vi "Stop.vi"(8 "error in (no error)":errorcluster, 10 "Message in":refnum<class "StopMessage.lvclass">, 11 "DAQMH121119OrcaFlash in":refnum<class "DAQOrcaFlash.lvclass">) -> (0 "error out":errorcluster, 3 "DAQMH121119OrcaFlash out":refnum<class "DAQOrcaFlash.lvclass">)   [LabVIEW 2012, in "DAQOrcaFlash.lvclass"]
doc: "This member function is called when the statemachine in the run.vi receives an 'stop' command. It relays the message to all observers of the component.\n\nOverride this member function in your derived class if you need additional stop functionality (but don't forget to call the parent method)."
uses:
  DAQOrcaFlash.lvclass
  <vilib>/Distrio/Murmex/StopMessage/StopMessage.lvclass
  <vilib>/Distrio/Murmex/Murmex/Murmex.lvclass
  trigger_source.ctl
  trigger_mode.ctl
  DAQOrcaFlash.lvclass/DAQOrcaFlash.ctl
  imaging_mode.ctl
panel:
  # "This method is called when the STOP\ntrigger is sent. \n\nOverride this method when your component needs to\nrespond to this trigger. \n\nCall parent for proper implementation"
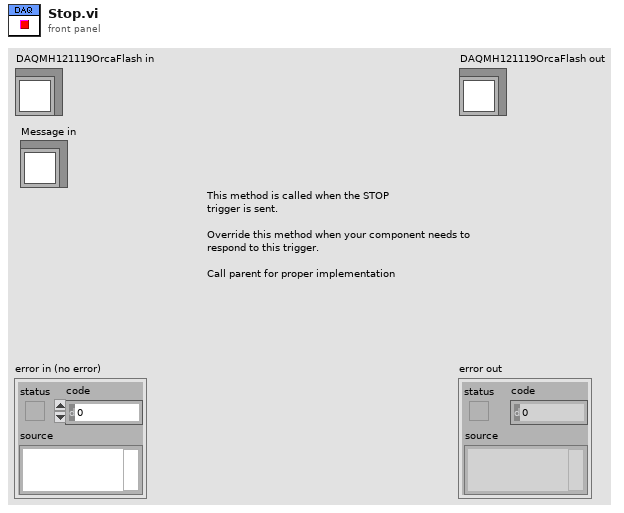
[diagram p1: front panel]
types:
  T1 = typedef "DAQOrcaFlash.lvclass/imaging_mode.ctl" = enum16{"focus mode", "single sweep"}
  T2 = typedef "DAQOrcaFlash.lvclass/trigger_mode.ctl" = sgl
  T3 = typedef "DAQOrcaFlash.lvclass/trigger_source.ctl" = sgl
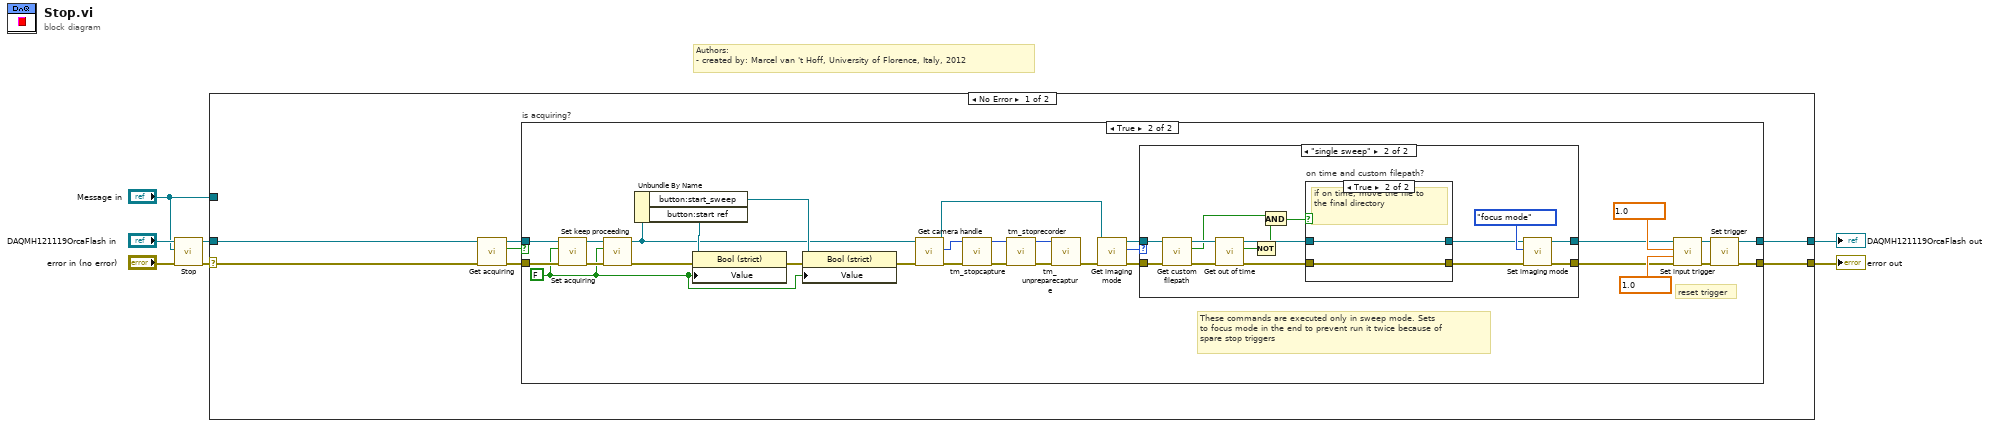
[diagram p0: block diagram]
diagram:
  # "Authors: \n- created by: Marcel van 't Hoff, University of Florence, Italy, 2012"
  n1 = call-parent "Stop.vi"("error in (no error)"="error in (no error)", "Message in"="Message in", "Murmex in"="DAQMH121119OrcaFlash in") -> ("error out"=w5:errorcluster, "Murmex out"=w2:refnum<class "DAQOrcaFlash.lvclass">)  [unwired: 7 in]
  n2 = case shown="No Error" w5 {
    selector: w5 -> [w9 w68]
    tunnel: [w11 w68] -> w4
    tunnel: [w10 w69] -> w3
    tunnel: w2 -> [w8 w69]
    tunnel: "Message in" -> [_ _]
    frame No Error {
      n3 = call "Get acquiring.vi"("error in (no error)"=w9, "DAQMH121119OrcaFlash in"=w8) -> ("error out"=w13:errorcluster, "is acquiring?"=w12:bool, "DAQMH121119OrcaFlash out"=w14:refnum<class "DAQOrcaFlash.lvclass">)  [unwired: 7 in]
      n4 = case "is acquiring?" shown="True" w12 {
        tunnel: [w15 w17] -> w10
        tunnel: [w16 w19] -> w11
        tunnel: w14 -> [w15 w44]
        tunnel: w13 -> [w16 w43]
        frame False {
        }
        frame True {
          w21 = T2 1.0 items=["Normal"=1.0, "Start"=6.0] ("Trigger mode")
          w22 = T3 1.0 items=["Internal"=1.0, "External"=2.0, "Software"=3.0] ("Trigger source")
          w25 = FALSE ("is acquiring?")
          # "reset trigger"
          # "These commands are executed only in sweep mode. Sets\nto focus mode in the end to prevent run it twice because of \nspare stop triggers"
          n5 = call "Set acquiring.vi"("error in (no error)"=w43, "is acquiring?"=w25, "DAQMH121119OrcaFlash in"=w44) -> ("error out"=w45:errorcluster, "DAQMH121119OrcaFlash out"=w27:refnum<class "DAQOrcaFlash.lvclass">)  [unwired: 7 in]
          n6 = call-dynamic "Set keep proceeding.vi"("error in (no error)"=w45, "keep proceeding?"=w25, "DAQOrcaFlash in"=w27) -> ("error out"=w28:errorcluster, "DAQOrcaFlash out"=w26:refnum<class "DAQOrcaFlash.lvclass">)  [unwired: 7 in]
          n7 = Unbundle By Name(w26) -> ("button:start_sweep"=w42:refnum<vi>, "button:start ref"=w46:refnum<vi>)
          n8 = property class="Bool (strict)"(reference=w46, error in=w28, "Value"=w25) -> (error out=w41:errorcluster)  [unwired: 1 out]
          n9 = property class="Bool (strict)"(reference=w42, error in=w41, "Value"=w25) -> (error out=w40:errorcluster)  [unwired: 1 out]
          n10 = call "Get camera handle.vi"("error in (no error)"=w40, "DAQMH121119OrcaFlash in"=w26) -> ("error out"=w32:errorcluster, "cam handle"=w31:u32, "DAQMH121119OrcaFlash out"=w37:refnum<class "DAQOrcaFlash.lvclass">)  [unwired: 7 in]
          n11 = call <userlib>:"tm_stopcapture.vi"("error in (no error)"=w32, "Handle in"=w31) -> ("error out"=w33:errorcluster, "Handle out"=w30:u32)  [unwired: 8 in]
          n12 = call <userlib>:"tm_stoprecorder.vi"("error in (no error)"=w33, "Handle in"=w30) -> ("error out"=w34:errorcluster, "Handle out"=w29:u32)  [unwired: 8 in]
          n13 = call <userlib>:"tm_unpreparecapture.vi"("error in (no error)"=w34, "Handle in"=w29) -> ("error out"=w39:errorcluster)  [unwired: 8 in, 1 out]
          n14 = call "Get imaging mode.vi"("error in (no error)"=w39, "DAQMH121119OrcaFlash in"=w37) -> ("error out"=w38:errorcluster, "imaging mode"=w35:T1, "DAQMH121119OrcaFlash out"=w36:refnum<class "DAQOrcaFlash.lvclass">)  [unwired: 7 in]
          n15 = case shown="\"single sweep\"" w35 {
            tunnel: w38 -> [w47 w56]
            tunnel: [w47 w63] -> w20
            tunnel: [w48 w62] -> w18
            tunnel: w36 -> [w48 w54]
            frame "focus mode", Default {
            }
            frame "single sweep" {
              n16 = call-dynamic "Get custom filepath.vi"("error in (no error)"=w56, "DAQOrcaFlash in"=w54) -> ("error out"=w55:errorcluster, "Custom saving path"=w50:bool, "DAQOrcaFlash out"=w53:refnum<class "DAQOrcaFlash.lvclass">)  [unwired: 7 in]
              n17 = call-dynamic "Get out of time.vi"("error in (no error)"=w55, "DAQOrcaFlash in"=w53) -> ("error out"=w57:errorcluster, "out of time?"=w52:bool, "DAQOrcaFlash out"=w58:refnum<class "DAQOrcaFlash.lvclass">)  [unwired: 7 in]
              n18 = Not(x=w52) -> (.not. x?=w51:bool)
              n19 = And(x=w50, y=w51) -> (x .and. y?=w49:bool)
              n20 = case "on time and custom filepath?" shown="True" w49 {
                tunnel: w57 -> [w64 w66]
                tunnel: [w64 w66] -> w60
                tunnel: w58 -> [w65 w67]
                tunnel: [w65 w67] -> w59
                frame False {
                  # "if out of time do nothing"
                }
                frame True {
                  # "if on time, move the file to\nthe final directory"
                }
              }
              n21 = call "Set imaging mode.vi"("error in (no error)"=w60, "imaging mode"=imaging_mode."focus mode", "DAQMH121119OrcaFlash in"=w59) -> ("error out"=w63:errorcluster, "DAQMH121119OrcaFlash out"=w62:refnum<class "DAQOrcaFlash.lvclass">)  [unwired: 7 in]
            }
          }
          n22 = call-dynamic "Set input trigger.vi"("error in (no error)"=w20, "Trigger mode"=w21, "Trigger source"=w22, "DAQOrcaFlash in"=w18) -> ("error out"=w23:errorcluster, "DAQOrcaFlash out"=w24:refnum<class "DAQOrcaFlash.lvclass">)  [unwired: 6 in]
          n23 = call-dynamic "Set trigger.vi"("error in (no error)"=w23, "DAQOrcaFlash in"=w24) -> ("error out"=w19:errorcluster, "DAQOrcaFlash out"=w17:refnum<class "DAQOrcaFlash.lvclass">)  [unwired: 8 in]
        }
      }
    }
    frame Error {
    }
  }
  "error out" <- w4
  "DAQMH121119OrcaFlash out" <- w3
